vi "Data Logger.vi"(10 "logging rate (ms)":u32, 11 "YOU WANT TO LOG?":bool) -> ()   [LabVIEW 2016]
uses:
  Globale Variablen VI/AutonomousMode.vi
  Globale Variablen VI/Logging Globale Variable.vi
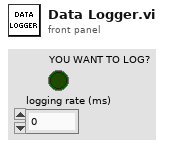
[diagram p1: front panel]
types:
  T1 = enum16{"open", "replace", "create", "open or create", "replace or create", "replace or create with confirmation"}
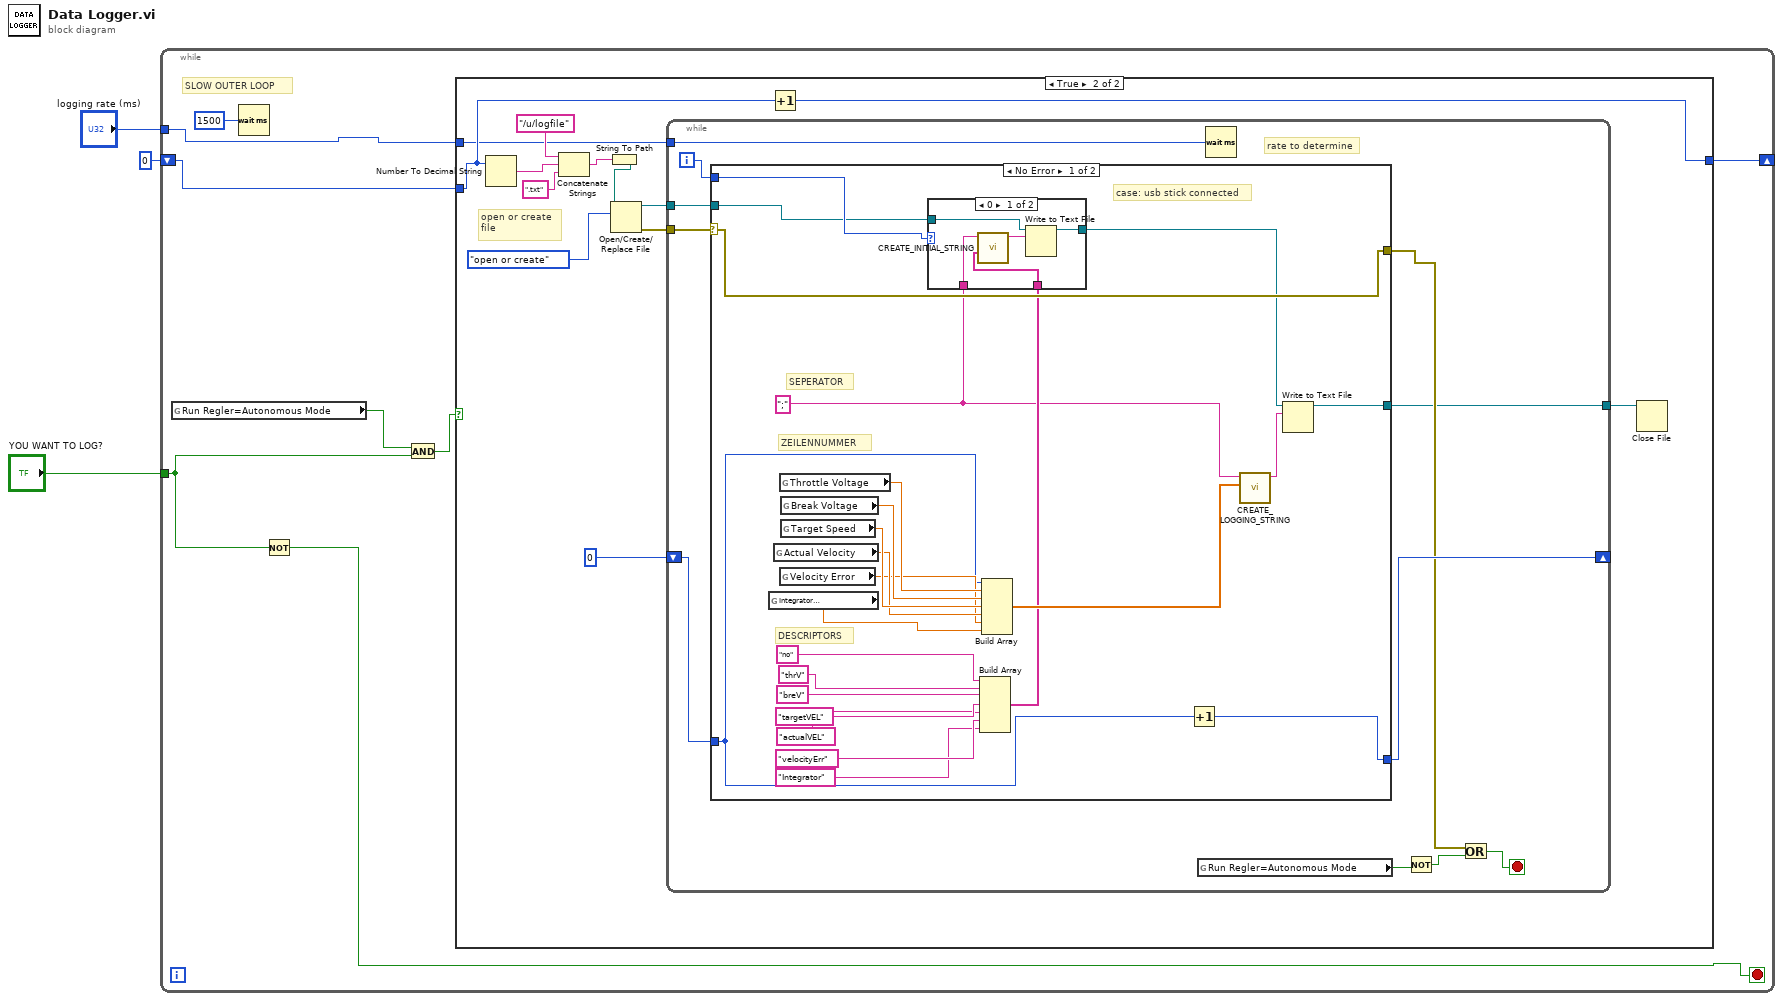
[diagram p0: block diagram]
diagram:
  n1 = while {
    shift-right: [w10] -> _
    shift-left: i16 0 -> [w9]
    tunnel: "YOU WANT TO LOG?" -> [w6]
    tunnel: "logging rate (ms)" -> [w4]
    stop <- w5 stop-if-true
    # "SLOW OUTER LOOP"
    n2 = global read "AutonomousMode.vi" "Run Regler=Autonomous Mode"() -> (w8:bool)
    n3 = Wait (ms)(milliseconds to wait=u32 1500) -> ()  [unwired: 1 out]
    n4 = Not(x=w6) -> (.not. x?=w5:bool)
    n5 = And(x=w8, y=w6) -> (x .and. y?=w7:bool)
    n6 = case shown="True" w7 {
      tunnel: w9 -> [w12 w19]
      tunnel: [w12 w18] -> w10
      tunnel: w4 -> [_ w13]
      frame False {
      }
      frame True {
        # "open or create \nfile"
        n7 = Number To Decimal String(number=w19) -> (decimal integer string=w15:string)  [unwired: 1 in]
        n8 = Concatenate Strings("/u/logfile" ("string"), w15, ".txt") -> (w16:string)
        n9 = String To Path(string=w16) -> (path=w23:path)
        n10 = Open/Create/Replace File(file path (use dialog)=w23, operation (0:open)=T1."open or create") -> (refnum out=w21:refnum<file>, error out=w22:errorcluster)  [unwired: 4 in, 1 out]
        n11 = while {
          shift-right: [w33] -> _
          shift-left: i16 0 ("width (-)") -> [w35]
          tunnel: w22 -> [w36]
          tunnel: w21 -> [w34]
          tunnel: [w30] -> w20
          tunnel: w13 -> [w28]
          i -> [w29]
          stop <- w32 stop-if-true
          # "rate to determine"
          n12 = case shown="No Error" w36 {
            selector: w36 -> [w51 w68]
            tunnel: [w51 w68] -> w31
            tunnel: w35 -> [w52 w69]
            tunnel: [w60 w69] -> w33
            tunnel: w34 -> [w42 w67]
            tunnel: [w50 w67] -> w30
            tunnel: w29 -> [w43 _]
            frame No Error {
              w39 = ";"
              # "DESCRIPTORS"
              # "ZEILENNUMMER"
              # "SEPERATOR"
              # "case: usb stick connected"
              n13 = global read "Logging Globale Variable.vi" "Integrator\nValue"() -> (w38:dbl)
              n14 = global read "Logging Globale Variable.vi" "Actual Velocity"() -> (w56:dbl)
              n15 = global read "Logging Globale Variable.vi" "Throttle Voltage"() -> (w59:dbl)
              n16 = global read "Logging Globale Variable.vi" "Velocity Error"() -> (w55:dbl)
              n17 = global read "Logging Globale Variable.vi" "Break Voltage"() -> (w58:dbl)
              n18 = global read "Logging Globale Variable.vi" "Target Speed"() -> (w57:dbl)
              n19 = Build Array("no", "thrV", "breV", "targetVEL", "actualVEL", "velocityErr", "Integrator") -> (w40:string[])
              n20 = case shown="0" w43 {
                tunnel: w42 -> [w65 w66]
                tunnel: [w64 w66] -> w41
                tunnel: w39 -> [w63 _]
                tunnel: w40 -> [w61 _]
                frame 0 {
                  n21 = call "CREATE_INITIAL_STRING.vi"("appended array"=w61, "String in"=w63) -> ("String out"=w62:string)  [unwired: 9 in]
                  n22 = Write to Text File(file (use dialog)=w65, text=w62) -> (refnum out=w64:refnum<file>)  [unwired: 2 in, 2 out]
                }
                frame Default {
                }
              }
              n23 = Build Array(w52, w59, w58, w57, w56, w55, w38) -> (w54:dbl[])
              n24 = Increment(x=w52) -> (x+1=w60:i16)
              n25 = call "CREATE_LOGGING_STRING.vi"("Array"=w54, "String in"=w39) -> ("String out"=w53:string)  [unwired: 9 in]
              n26 = Write to Text File(file (use dialog)=w41, text=w53) -> (refnum out=w50:refnum<file>)  [unwired: 2 in, 2 out]
            }
            frame Error {
              # "case: no usb stick connected"
            }
          }
          n27 = global read "AutonomousMode.vi" "Run Regler=Autonomous Mode"() -> (w27:bool)
          n28 = Wait (ms)(milliseconds to wait=w28) -> ()  [unwired: 1 out]
          n29 = Not(x=w27) -> (.not. x?=w26:bool)
          n30 = Or(x=w31, y=w26) -> (x .or. y?=w32:bool)
        }
        n31 = Increment(x=w19) -> (x+1=w18:i16)
        n32 = Close File(refnum=w20) -> ()  [unwired: 1 in, 2 out]
      }
    }
  }
